vi "display_michelle_visjitter_stopadded_RandCont_Psuedo_FrameClock.vi"() -> ()   [LabVIEW 2019]
uses:
  <vilib>/Analysis/Matrix/Datatypes/RealMatrix.ctl
  <vilib>/Utility/file.llb/Write Delimited Spreadsheet (DBL).vi
  <vilib>/Analysis/Matrix/NI_Matrix.lvlib
panel:
  out "lambda":dbl
  out "maxITI":dbl
  out "minITII":dbl
  out "goEXP":dbl
  out "ArrayTemp3":T1
  out "StimID2":dbl
  out "Contrast":dbl
  out "TimeOutCounter":i32
  out "ElapsedTime_M":dbl
  out "Base_Contrast":dbl
  out "CurrentTrial":u32=1
  out "Jitter":dbl
  out "BaseITI":dbl
  out "VisStimDuration":dbl
  in  "Stop":bool
  out "Num trials":u32=204
  out "ISI Time":dbl
  out "Stim TS":dbl
  out "Output":dbl[][](array[numeric])
  out "Output frame":T1
  out "Array temp1":T1
  out "Elapsed Time":dbl
  out "Display":bool=TRUE
  out "Trial":u32=1
  out "reward":dbl[](array[numeric])
  out "stim_id":dbl[](array[numeric])
  out "stim_loaded":dbl
  out "Timings":dbl[](array[numeric])
  out "Stimuli Loaded?":bool
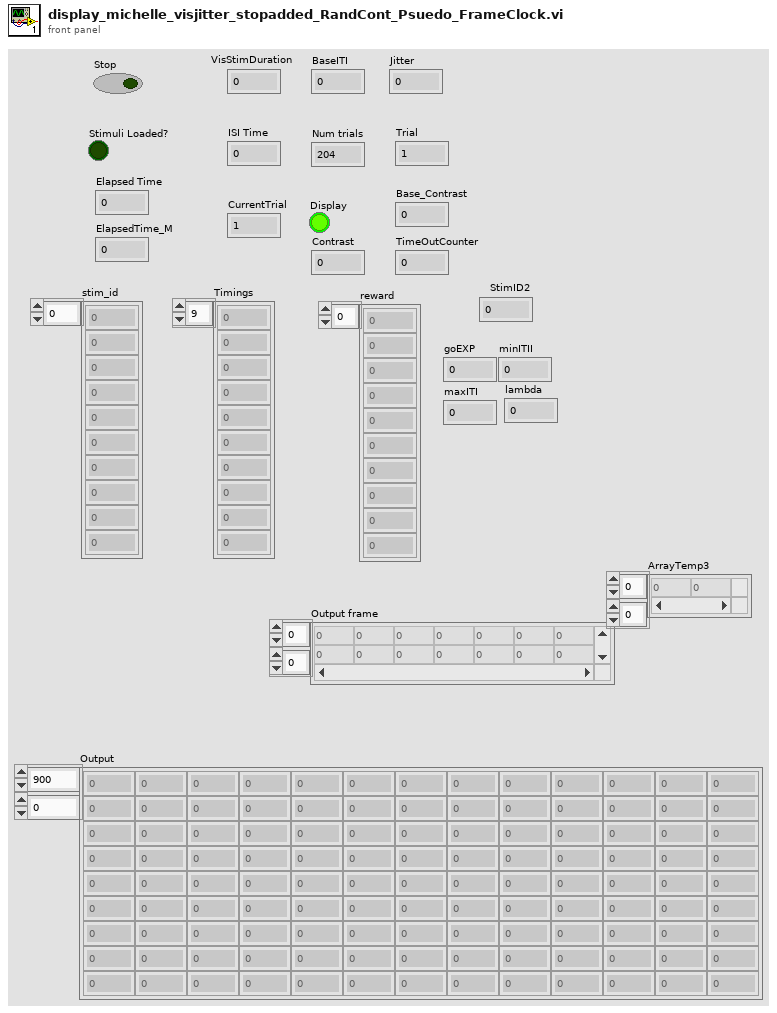
[diagram p1: front panel]
types:
  T1 = typedef "NI_Matrix.lvlib/RealMatrix.ctl" = dbl[][]
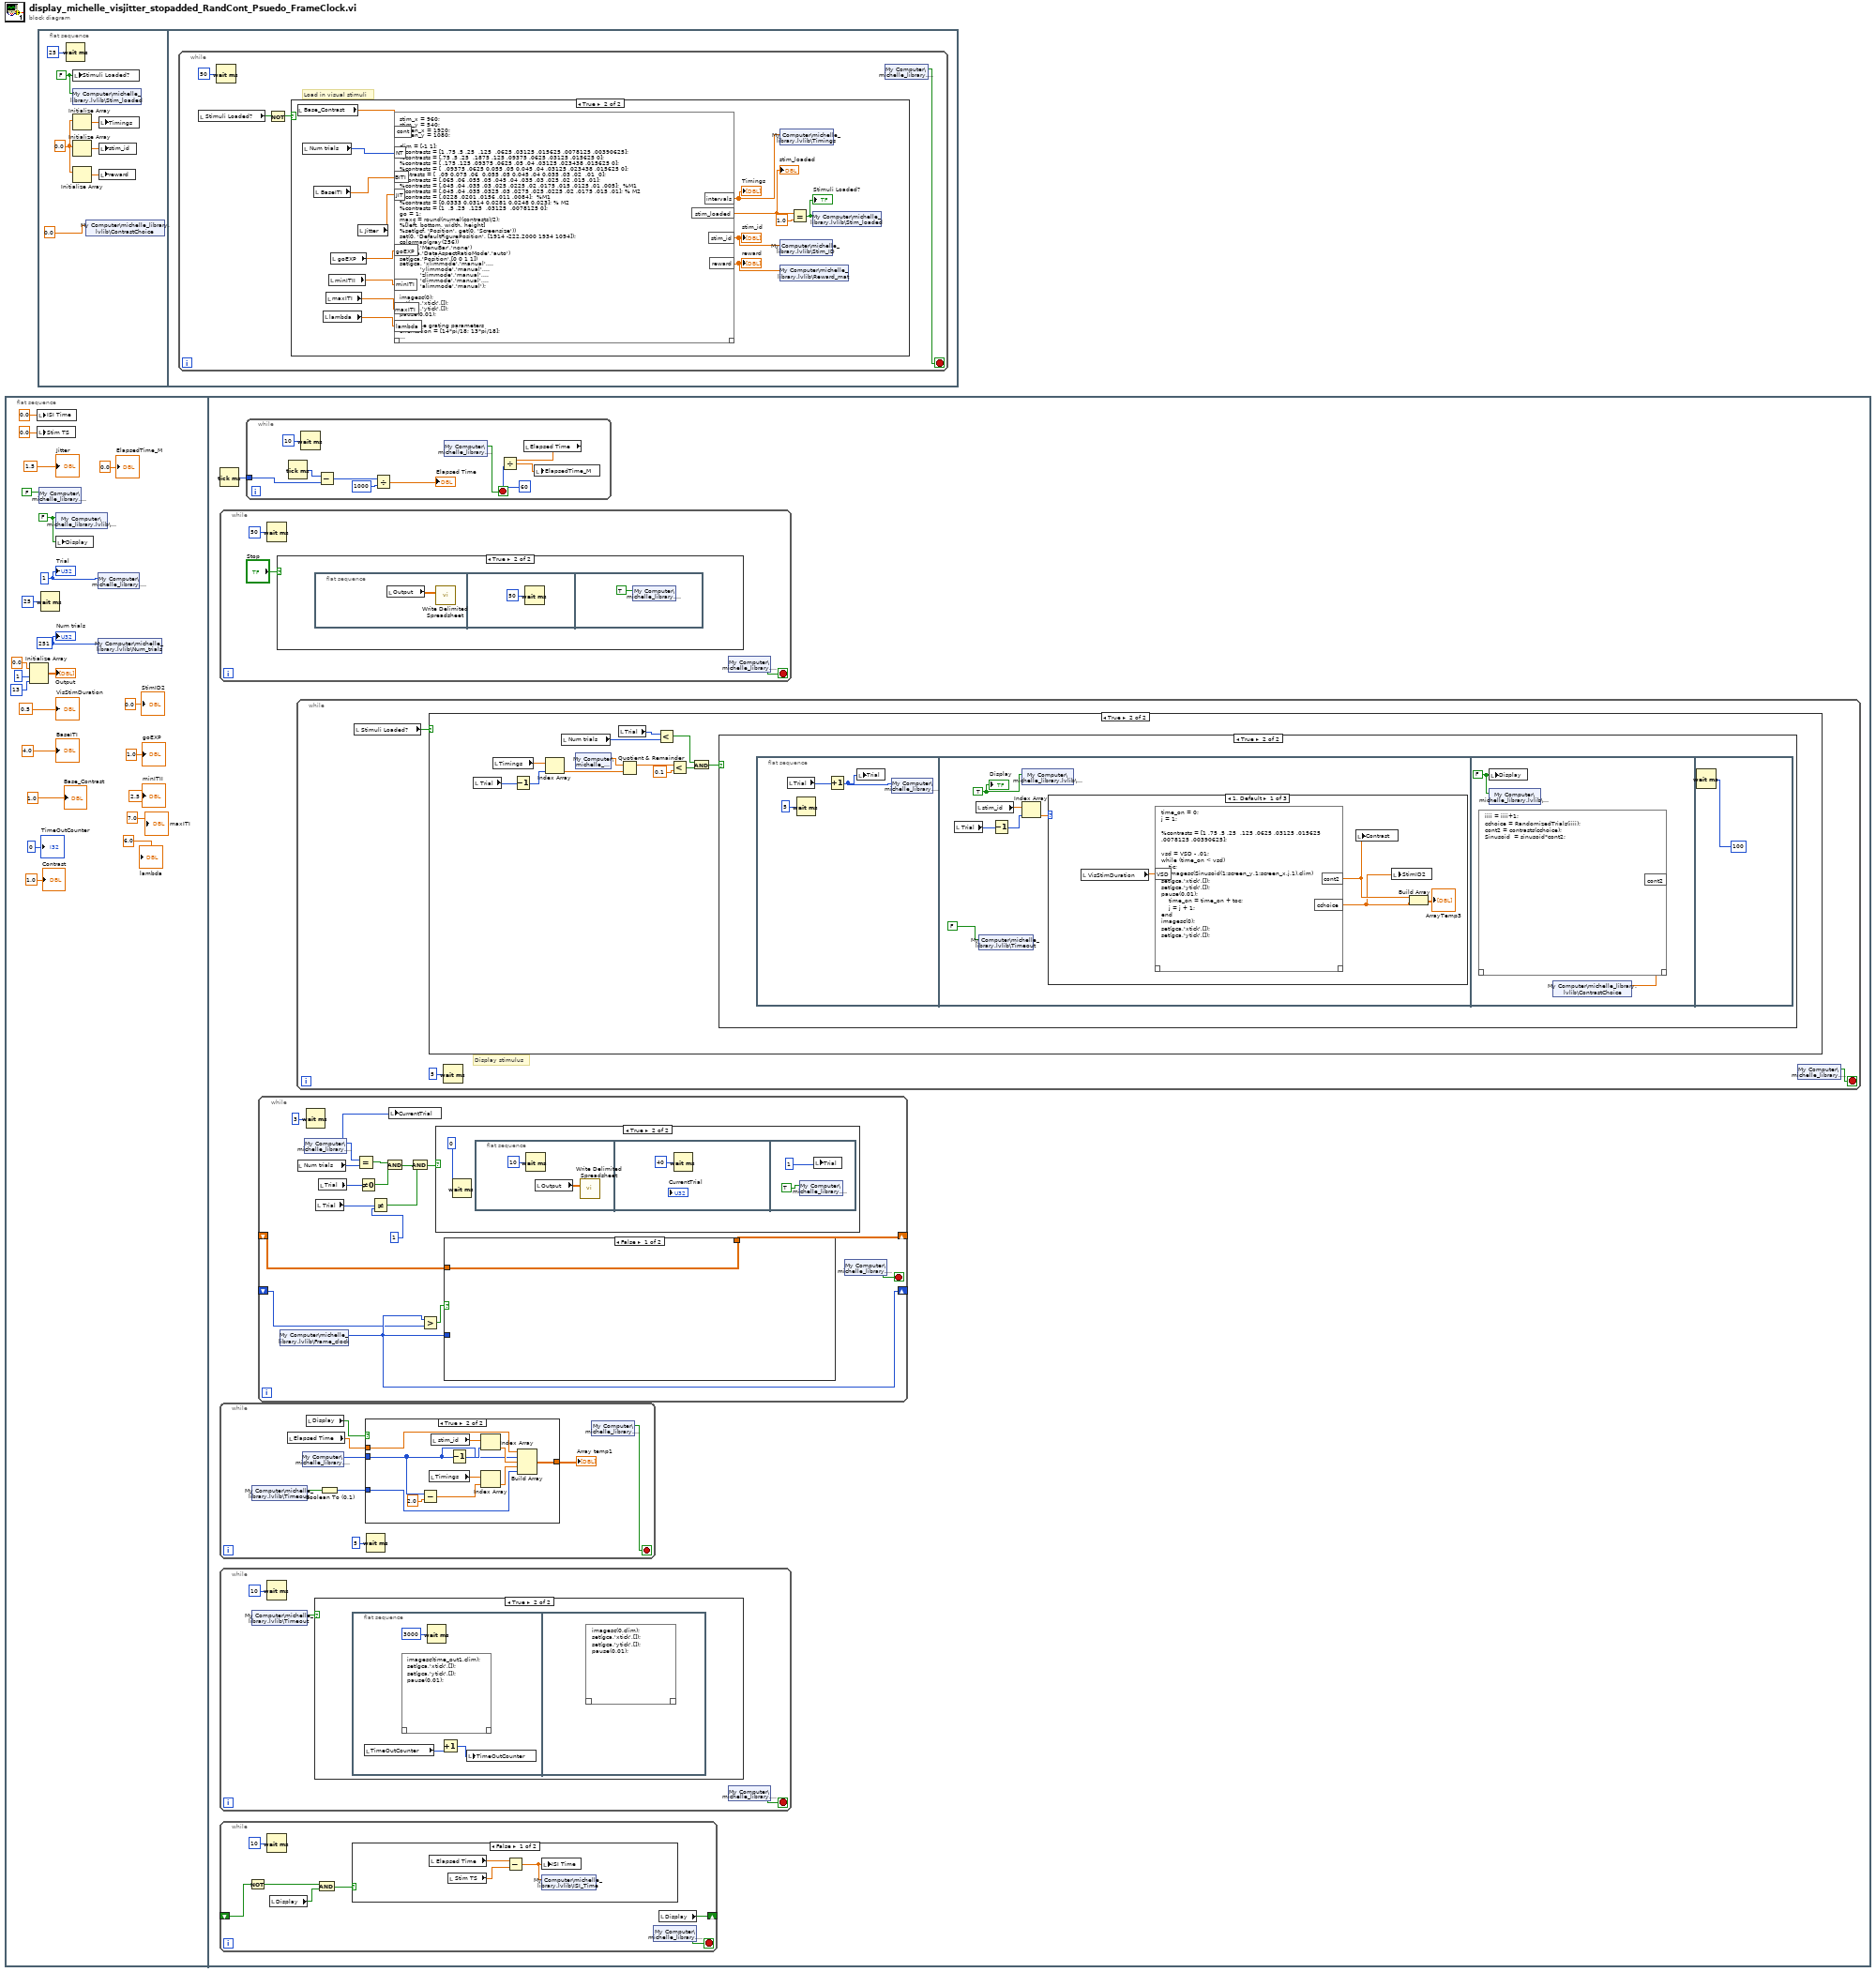
[diagram p0: block diagram]
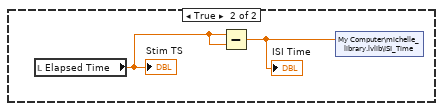
[diagram p5: hidden frame]
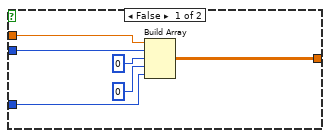
[diagram p6: hidden frame]
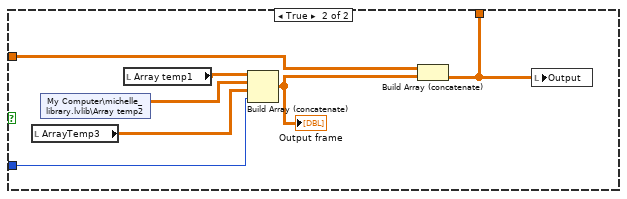
[diagram p7: hidden frame]
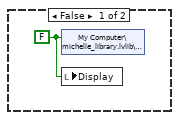
[diagram p10: hidden frame]
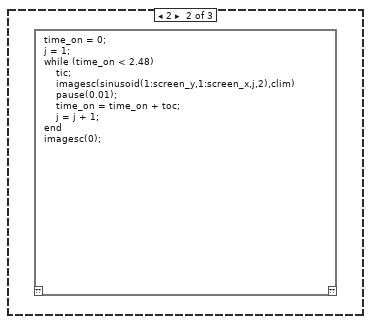
[diagram p11: hidden frame]
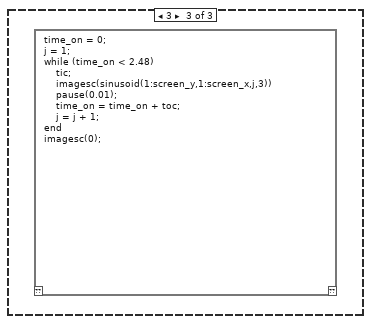
[diagram p12: hidden frame]
diagram:
  n1 = flat-sequence {
    frame #0 {
      w15 = u32 251
      w21 = FALSE ("Display")
      w23 = u32 1 ("Trial")
      n2 = Initialize Array(0.0 ("element"), 1 ("dimension size"), 13 ("dimension size")) -> (→"Output":dbl[][])
      n3 = local write "ISI Time"(0.0 ("ISI Time")) -> ()
      n4 = local write "Stim TS"(0.0 ("Stim TS")) -> ()
      n5 = shared-variable "My Computer\\michelle_library.lvlib\\Stop"(FALSE ("Stop")) -> ()  [unwired: 1 in, 1 out]
      n6 = Wait (ms)(milliseconds to wait=u32 25) -> ()  [unwired: 1 out]
      n7 = shared-variable "My Computer\\michelle_library.lvlib\\Display"(w21) -> ()  [unwired: 1 in, 1 out]
      n8 = local write "Display"(w21) -> ()
      n9 = shared-variable "My Computer\\michelle_library.lvlib\\Trial"(w23) -> ()  [unwired: 1 in, 1 out]
      n10 = shared-variable "My Computer\\michelle_library.lvlib\\Num_trials"(w15) -> ()  [unwired: 1 in, 1 out]
      "Trial" <- w23
      "Num trials" <- w15
      "VisStimDuration" <- 0.5
      "BaseITI" <- 4.0
      "Jitter" <- 1.5
      "Base_Contrast" <- 1.0
      "ElapsedTime_M" <- 0.0
      "TimeOutCounter" <- 0
      "Contrast" <- 1.0
      "StimID2" <- 0.0
      "goEXP" <- 1.0
      "minITII" <- 2.5
      "maxITI" <- 7.0
      "lambda" <- 6.0
    }
    frame #1 {
      n11 = Tick Count (ms)() -> (millisecond timer value=w24:u32)
      n12 = while {
        stop <- w27 stop-if-true
        n13 = Wait (ms)(milliseconds to wait=50) -> ()  [unwired: 1 out]
        n14 = case shown="True" "Stop" {
          frame False {
          }
          frame True {
            n15 = flat-sequence {
              frame #0 {
                n16 = local read "Output"() -> (w28:dbl[][])
                n17 = call-poly <vilib>:"Write Delimited Spreadsheet.vi"("2D data"=w28) -> ()  [unwired: 13 in, 2 out]
              }
              frame #1 {
                n18 = Wait (ms)(milliseconds to wait=50) -> ()  [unwired: 1 out]
              }
              frame #2 {
                n19 = shared-variable "My Computer\\michelle_library.lvlib\\Stop"(TRUE) -> ()  [unwired: 1 in, 1 out]
              }
            }
          }
        }
        n20 = shared-variable "My Computer\\michelle_library.lvlib\\Stop"() -> (w27:bool)  [unwired: 1 in, 1 out]
      }
      n21 = while {
        stop <- w51 stop-if-true
        n22 = shared-variable "My Computer\\michelle_library.lvlib\\Timeout"() -> (w49:bool)  [unwired: 1 in, 1 out]
        n23 = local read "Elapsed Time"() -> (w55:dbl)
        n24 = shared-variable "My Computer\\michelle_library.lvlib\\Trial"() -> (w53:u32)  [unwired: 1 in, 1 out]
        n25 = local read "Display"() -> (w52:bool)
        n26 = Boolean To (0,1)(Boolean=w49) -> (0, 1=w50:i16)
        n27 = case shown="True" w52 {
          tunnel: w53 -> [w61 w64]
          tunnel: w55 -> [w62 w71]
          tunnel: [w60 w72] -> w54
          tunnel: w50 -> [w57 w66]
          frame False {
            n28 = Build Array(w62, w61, u32 0 ("milliseconds to wait"), 0, w57) -> (w60:T1)
          }
          frame True {
            n29 = Subtract(x=w64, y=2.0) -> (x-y=w63:dbl)
            n30 = local read "Timings"() -> (w69:dbl[])
            n31 = local read "stim_id"() -> (w73:dbl[])
            n32 = Decrement(x=w64) -> (x-1=w68:u32)
            n33 = Index Array(array=w73, index=w68) -> (element=w70:dbl)
            n34 = Index Array(array=w69, index=w63) -> (element=w67:dbl)
            n35 = Build Array(w71, w64, w70, w67, w66) -> (w72:T1)
          }
        }
        "Array temp1" <- w54
        n36 = Wait (ms)(milliseconds to wait=u32 5) -> ()  [unwired: 1 out]
        n37 = shared-variable "My Computer\\michelle_library.lvlib\\Stop"() -> (w51:bool)  [unwired: 1 in, 1 out]
      }
      n38 = while {
        stop <- w33 stop-if-true
        n39 = shared-variable "My Computer\\michelle_library.lvlib\\Timeout"() -> (w31:bool)  [unwired: 1 in, 1 out]
        n40 = Wait (ms)(milliseconds to wait=u32 10) -> ()  [unwired: 1 out]
        n41 = case shown="True" w31 {
          frame False {
          }
          frame True {
            n42 = flat-sequence {
              frame #0 {
                n43 = local read "TimeOutCounter"() -> (w35:i32)
                n44 = script code="imagesc(time_out1,clim);\nset(gca,'xtick',[]);\nset(gca,'ytick',[]);\npause(0.01);"() -> ()  [unwired: 1 in, 1 out]
                n45 = Wait (ms)(milliseconds to wait=u32 3000) -> ()  [unwired: 1 out]
                n46 = Increment(x=w35) -> (x+1=w34:i32)
                n47 = local write "TimeOutCounter"(w34) -> ()
              }
              frame #1 {
                n48 = script code="imagesc(0,clim);\nset(gca,'xtick',[]);\nset(gca,'ytick',[]);\npause(0.01);"() -> ()  [unwired: 1 in, 1 out]
              }
            }
          }
        }
        n49 = shared-variable "My Computer\\michelle_library.lvlib\\Stop"() -> (w33:bool)  [unwired: 1 in, 1 out]
      }
      n50 = while {
        shift-right: [w41] -> _
        shift-left: _ -> [w40]
        stop <- w43 stop-if-true
        n51 = Not(x=w40) -> (.not. x?=w39:bool)
        n52 = Wait (ms)(milliseconds to wait=u32 10) -> ()  [unwired: 1 out]
        n53 = local read "Display"() -> (w38:bool)
        n54 = And(x=w39, y=w38) -> (x .and. y?=w37:bool)
        n55 = case shown="False" w37 {
          frame False {
            n56 = local read "Elapsed Time"() -> (w44:dbl)
            n57 = local read "Stim TS"() -> (w46:dbl)
            n58 = Subtract(x=w44, y=w46) -> (x-y=w45:dbl)
            n59 = local write "ISI Time"(w45) -> ()
            n60 = shared-variable "My Computer\\michelle_library.lvlib\\ISI_Time"(w45) -> ()  [unwired: 1 in, 1 out]
          }
          frame True {
            n61 = local read "Elapsed Time"() -> (w47:dbl)
            "Stim TS" <- w47
            n62 = Subtract(x=w47, y=w47) -> (x-y=w48:dbl)
            "ISI Time" <- w48
            n63 = shared-variable "My Computer\\michelle_library.lvlib\\ISI_Time"(w48) -> ()  [unwired: 1 in, 1 out]
          }
        }
        n64 = shared-variable "My Computer\\michelle_library.lvlib\\Stop"() -> (w43:bool)  [unwired: 1 in, 1 out]
        n65 = local read "Display"() -> (w41:bool)
      }
      n66 = while {
        tunnel: w24 -> [w80]
        stop <- w77 stop-if-true
        n67 = Tick Count (ms)() -> (millisecond timer value=w81:u32)
        n68 = Wait (ms)(milliseconds to wait=u32 10) -> ()  [unwired: 1 out]
        n69 = Subtract(x=w81, y=w80) -> (x-y=w78:u32)
        n70 = Divide(x=w78, y=u32 1000) -> (x/y=→"Elapsed Time":dbl)
        n71 = shared-variable "My Computer\\michelle_library.lvlib\\Stop"() -> (w77:bool)  [unwired: 1 in, 1 out]
        n72 = local read "Elapsed Time"() -> (w74:dbl)
        n73 = Divide(x=w74, y=60) -> (x/y=w76:dbl)
        n74 = local write "ElapsedTime_M"(w76) -> ()
      }
      n75 = while {
        shift-right: [w97] -> _
        shift-left: _ -> [w98]
        shift-right: [w87] -> _
        shift-left: _ -> [w86]
        stop <- w100 stop-if-true
        n76 = shared-variable "My Computer\\michelle_library.lvlib\\Frame_clock"() -> (w87:u32)  [unwired: 1 in, 1 out]
        n77 = local read "Num trials"() -> (w96:u32)
        n78 = shared-variable "My Computer\\michelle_library.lvlib\\Trial"() -> (w88:u32)  [unwired: 1 in, 1 out]
        n79 = Wait (ms)(milliseconds to wait=u32 3) -> ()  [unwired: 1 out]
        n80 = local read "Trial"() -> (w93:u32)
        n81 = local read "Trial"() -> (w94:u32)
        n82 = Equal?(x=w88, y=w96) -> (x = y?=w95:bool)
        n83 = Not Equal To 0?(x=w94) -> (x != 0?=w91:bool)
        n84 = Not Equal?(x=w93, y=1) -> (x != y?=w92:bool)
        n85 = And(x=w95, y=w91) -> (x .and. y?=w89:bool)
        n86 = local write "CurrentTrial"(w88) -> ()
        n87 = And(x=w89, y=w92) -> (x .and. y?=w90:bool)
        n88 = Greater?(x=w87, y=w86) -> (0:w84:bool)
        n89 = case shown="True" w90 {
          frame False {
          }
          frame True {
            n90 = Wait (ms)(milliseconds to wait=0) -> ()  [unwired: 1 out]
            n91 = flat-sequence {
              frame #0 {
                n92 = Wait (ms)(milliseconds to wait=u32 10) -> ()  [unwired: 1 out]
                n93 = local read "Output"() -> (w111:dbl[][])
                n94 = call-poly <vilib>:"Write Delimited Spreadsheet.vi"("2D data"=w111) -> ()  [unwired: 13 in, 2 out]
              }
              frame #1 {
                n95 = Wait (ms)(milliseconds to wait=u32 40) -> ()  [unwired: 1 out]
              }
              frame #2 {
                n96 = shared-variable "My Computer\\michelle_library.lvlib\\Stop"(TRUE) -> ()  [unwired: 1 in, 1 out]
                n97 = local write "Trial"(1) -> ()
              }
            }
          }
        }
        n98 = case shown="False" w84 {
          tunnel: w98 -> [w101 w108]
          tunnel: [w101 w107] -> w97
          tunnel: w87 -> [_ w102]
          frame False {
          }
          frame True {
            n99 = local read "ArrayTemp3"() -> (w103:T1)
            n100 = shared-variable "My Computer\\michelle_library.lvlib\\Array temp2"() -> (w105:dbl[][])  [unwired: 1 in, 1 out]
            n101 = local read "Array temp1"() -> (w106:T1)
            n102 = Build Array (concatenate)(w106, w105, w103, w102) -> (w104:T1)
            "Output frame" <- w104
            n103 = Build Array (concatenate) ("Build Matrix")(w108, w104) -> (w107:T1)
            n104 = local write "Output"(w107) -> ()
          }
        }
        n105 = shared-variable "My Computer\\michelle_library.lvlib\\Stop"() -> (w100:bool)  [unwired: 1 in, 1 out]
      }
      n106 = while {
        stop <- w116 stop-if-true
        # "Display stimulus"
        n107 = local read "Stimuli Loaded?"() -> (w115:bool)
        n108 = case shown="True" w115 {
          frame False {
          }
          frame True {
            n109 = local read "Trial"() -> (w118:u32)
            n110 = local read "Timings"() -> (w127:dbl[])
            n111 = Decrement(x=w118) -> (x-1=w119:u32)
            n112 = Index Array(array=w127, index=w119) -> (element=w126:dbl)
            n113 = local read "Num trials"() -> (w122:u32)
            n114 = shared-variable "My Computer\\michelle_library.lvlib\\ISI"() -> (w121:dbl)  [unwired: 1 in, 1 out]
            n115 = local read "Trial"() -> (w125:u32)
            n116 = Quotient & Remainder(x=w121, y=w126) -> (x-y*floor(x/y)=w129:dbl)  [unwired: 1 out]
            n117 = Less?(x=w125, y=w122) -> (x < y?=w124:bool)
            n118 = Less?(x=w129, y=0.1) -> (x < y?=w123:bool)
            n119 = And(x=w124, y=w123) -> (x .and. y?=w120:bool)
            n120 = case shown="True" w120 {
              frame False {
                w130 = FALSE ("Display")
                n121 = shared-variable "My Computer\\michelle_library.lvlib\\Display"(w130) -> ()  [unwired: 1 in, 1 out]
                n122 = local write "Display"(w130) -> ()
              }
              frame True {
                n123 = flat-sequence {
                  frame #0 {
                    n124 = local read "Trial"() -> (w133:u32)
                    n125 = Wait (ms)(milliseconds to wait=u32 5) -> ()  [unwired: 1 out]
                    n126 = Increment(x=w133) -> (x+1=w132:u32)
                    n127 = local write "Trial"(w132) -> ()
                    n128 = shared-variable "My Computer\\michelle_library.lvlib\\Trial"(w132) -> ()  [unwired: 1 in, 1 out]
                  }
                  frame #1 {
                    w138 = TRUE ("Boolean")
                    n129 = local read "Trial"() -> (w136:u32)
                    n130 = local read "stim_id"() -> (w139:dbl[])
                    n131 = shared-variable "My Computer\\michelle_library.lvlib\\Timeout"(FALSE) -> ()  [unwired: 1 in, 1 out]
                    n132 = Decrement(x=w136) -> (x-1=w135:u32)
                    n133 = shared-variable "My Computer\\michelle_library.lvlib\\Display"(w138) -> ()  [unwired: 1 in, 1 out]
                    n134 = Index Array(array=w139, index=w135) -> (element=w137:dbl)
                    n135 = case shown="1, Default" w137 {
                      frame 1, Default {
                        n136 = local read "VisStimDuration"() -> (w143:dbl)
                        n137 = script code="time_on = 0;\nj = 1;\n\n%contrasts = [1 .75 .5 .25  .125 .0625 .03125 .015625 .0078125 .00390625];\n\nvsd = VSD - .01;\nwhile (time_on < vsd)\n    tic;\n    imagesc(Sinusoid(1:screen_y,1:screen_x,j,1),clim)\nset(gca,'xtick',[]);\nset(gca,'ytick',[]);    \npause(0.01);\n    time_on = time_on + toc;\n    j = j + 1;\nend\nimagesc(0);\nset(gca,'xtick',[]);\nset(gca,'ytick',[]);"("VSD"=w143) -> ("cont2"=w142:dbl, "cchoice"=w141:dbl)  [unwired: 1 in, 1 out]
                        n138 = local write "Contrast"(w142) -> ()
                        n139 = local write "StimID2"(w141) -> ()
                        n140 = Build Array(w142, w141) -> (→"ArrayTemp3":T1)
                      }
                      frame 2 {
                        n141 = script code="time_on = 0;\nj = 1;\nwhile (time_on < 2.48)\n    tic;\n    imagesc(sinusoid(1:screen_y,1:screen_x,j,2),clim)\n    pause(0.01);\n    time_on = time_on + toc;\n    j = j + 1;\nend\nimagesc(0);"() -> ()  [unwired: 1 in, 1 out]
                      }
                      frame 3 {
                        n142 = script code="time_on = 0;\nj = 1;\nwhile (time_on < 2.48)\n    tic;\n    imagesc(sinusoid(1:screen_y,1:screen_x,j,3))\n    pause(0.01);\n    time_on = time_on + toc;\n    j = j + 1;\nend\nimagesc(0);"() -> ()  [unwired: 1 in, 1 out]
                      }
                    }
                    "Display" <- w138
                  }
                  frame #2 {
                    w145 = FALSE ("Display")
                    n143 = script code="iiii = iiii+1;\ncchoice = RandomizedTrials(iiii);\ncont2 = contrasts(cchoice);\nSinusoid  = sinusoid*cont2;"() -> ("cont2"=w144:dbl)  [unwired: 1 in, 1 out]
                    n144 = local write "Display"(w145) -> ()
                    n145 = shared-variable "My Computer\\michelle_library.lvlib\\Display"(w145) -> ()  [unwired: 1 in, 1 out]
                    n146 = shared-variable "My Computer\\michelle_library.lvlib\\ContrastChoice"(w144) -> ()  [unwired: 1 in, 1 out]
                  }
                  frame #3 {
                    n147 = Wait (ms)(milliseconds to wait=u32 100) -> ()  [unwired: 1 out]
                  }
                }
              }
            }
          }
        }
        n148 = Wait (ms)(milliseconds to wait=u32 5) -> ()  [unwired: 1 out]
        n149 = shared-variable "My Computer\\michelle_library.lvlib\\Stop"() -> (w116:bool)  [unwired: 1 in, 1 out]
      }
    }
  }
  n150 = flat-sequence {
    frame #0 {
      w150 = 0.0 ("element")
      w148 = FALSE ("Stimuli Loaded?")
      n151 = Wait (ms)(milliseconds to wait=u32 25) -> ()  [unwired: 1 out]
      n152 = local write "Stimuli Loaded?"(w148) -> ()
      n153 = shared-variable "My Computer\\michelle_library.lvlib\\Stim_loaded"(w148) -> ()  [unwired: 1 in, 1 out]
      n154 = Initialize Array(w150) -> (w152:dbl[])  [unwired: 1 in]
      n155 = Initialize Array(w150) -> (w151:dbl[])  [unwired: 1 in]
      n156 = Initialize Array(w150) -> (w149:dbl[])  [unwired: 1 in]
      n157 = shared-variable "My Computer\\michelle_library.lvlib\\ContrastChoice"(0.0) -> ()  [unwired: 1 in, 1 out]
      n158 = local write "Timings"(w152) -> ()
      n159 = local write "stim_id"(w151) -> ()
      n160 = local write "reward"(w149) -> ()
    }
    frame #1 {
      n161 = while {
        stop <- w156 stop-if-true
        # "Load in visual stimuli"
        n162 = local read "Stimuli Loaded?"() -> (w155:bool)
        n163 = Wait (ms)(milliseconds to wait=u32 50) -> ()  [unwired: 1 out]
        n164 = Not(x=w155) -> (.not. x?=w154:bool)
        n165 = case shown="True" w154 {
          frame False {
          }
          frame True {
            n166 = local read "Base_Contrast"() -> (w162:dbl)
            n167 = local read "Num trials"() -> (w165:u32)
            n168 = local read "BaseITI"() -> (w164:dbl)
            n169 = local read "lambda"() -> (w161:dbl)
            n170 = local read "maxITI"() -> (w160:dbl)
            n171 = local read "minITII"() -> (w159:dbl)
            n172 = local read "goEXP"() -> (w158:dbl)
            n173 = local read "Jitter"() -> (w163:dbl)
            n174 = script code="stim_x = 960;\nstim_y = 540;\nscreen_x = 1920;\nscreen_y = 1080;\n\nclim = [-1 1];\n%contrasts = [1 .75 .5 .25  .125  .0625 .03125 .015625 .0078125 .00390625];\n%contrasts = [.75 .5 .25  .1875 .125 .09375 .0625 .03125 .015625 0];\n%contrasts = [ .175 .125 .09375 .0625 .05 .04 .03125 .023438 .015625 0];\n%contrasts = [  .09375 .0625 0.055 .05 0.045 .04 .03125 .023438 .015625 0];\ncontrasts = [  .09 0.075 .06  0.055 .05 0.045 .04 0.035 .03 .02  .01  0];\n%contrasts = [.065 .06 .055 .05 .045 .04 .035 .03 .025 .02 .015 .01];\n%contrasts = [.045 .04 .035 .03 .025 .0225 .02 .0175 .015 .0125 .01 .005];  %M1\n%contrasts = [.045 .04 .035 .0325 .03 .0275 .025 .0225 .02 .0175 .015 .01]; % M2\n%contrasts = [.0228 .0201 .0156 .011 .0084];  %M1\n%contrasts = [0.0333 0.0314 0.0281 0.0248 0.023]; % M2\n%contrasts = [1  .5 .25  .125  .03125  .0078125 0];\ngo = 1;\nmaxc = round(numel(contrasts)/2);\n%[left, bottom, width, height]\n%set(gcf, 'Position', get(0, 'Screensize'))\nset(0, 'DefaultFigurePosition', [1914 -222.2000 1934 1094]);\ncolormap(gray(256))\nset(gcf,'MenuBar','none')\nset(gca,'DataAspectRatioMode','auto')\nset(gca,'Position',[0 0 1 1])\nset(gca, 'xlimmode','manual',...\n           'ylimmode','manual',...\n           'zlimmode','manual',...\n           'climmode','manual',...\n           'alimmode','manual');\n\nimagesc(0);\nset(gca,'xtick',[]);\nset(gca,'ytick',[]);\npause(0.01);\n\n% Define grating parameters\norientation = [14*pi/18; 13*pi/18];\n\ncenter = [1,1]; %[0,0] is the middle of the image, [pi,pi] is the lower right\n%width = .5;  %1/e half width of Gaussian\nspatialFrequency = 8;  %spatial frequency of Sinewave carrier (cycles/image)\nphase = -pi/2; %spatial phase of sinewave carrier (radians)\ncontrast = cont;  %contrast ranges from 0 to 1;\n%screen_x = 1920; %resolution of the image  \n%screen_y = 1080;\n\n% Use meshgrid to define matrices X and Y that range from -pi to pi;\n[X,Y] = meshgrid(linspace(-pi,pi,screen_x),linspace(-pi/2,pi/2,screen_y));\n\nsinusoid = zeros(screen_y,screen_x,150,2);\ntime_out1 = ones(screen_y,screen_x)*-1;\ntime_out2 = zeros(screen_y,screen_x);\n%time_out(1,1) = 1;\n% Set up individual 4-d matrices (x, y, time, orientation) for movies of the drifting gratings at each\n% orientation\nfor j = 1:length(orientation)                                                            % Phase increase number here\n    ramp(1:screen_y,1:screen_x,j) = cos(orientation(j))*(X-center(1)) + sin(orientation(j))*(Y-center(2));     %  |\n    for i = 1:150 %Sets the number of frames to define gratings for                   V\n       sinusoid(1:screen_y,1:screen_x,i,j) = contrast*sin(spatialFrequency*ramp(1:screen_y,1:screen_x,j)-...\n           (phase+(2*pi*(i-1)*(-30)/360))); %Number before '/360' sets the phase increase\n    end\nend\n\n\n\n[RandomizedTrials]=RandomizeTrials_Psuedo_function(contrasts,NT,'n');\n\n\niiii = 1;\n\ncchoice = RandomizedTrials(iiii);\ncont2 = contrasts(cchoice);\nSinusoid  = sinusoid*cont2;\n\n\n%%  To be run of not using exponential\n%intervals = [ones(1,41)*10 ones(1,41)*11 ones(1,41)*12 ones(1,41)*13 ones(1,40)*14];\nif goEXP < 1\n     jit = JIT;\n     jitter = rand(1,NT);\n     jitter = 2*jit*(jitter- .5);\n     ITIbase = BITI;\n     intervals = [ones(1,NT)*ITIbase];\n     intervals = intervals + jitter;\nelseif goEXP > 0\n     intervals = exponentialITI(1/lambda, minITI, maxITI, NT);\nend\n%%\nstim_id = [ones(1,NT)*1];\n%reward = [ones(1,87)*1 ones(1,15)*0 ones(1,87)*1 ones(1,15)*0];\nreward = [ones(1,NT)*1];\n\n\n\nrand_idx1 = randperm(NT);\nrand_idx2 = randperm(NT);\nintervals = intervals(rand_idx2);\nstim_id = stim_id(rand_idx2);\nreward = reward(rand_idx2);\n\nstim_loaded = 1;" ("Script Node")("NT"=w165, "BITI"=w164, "JIT"=w163, "cont"=w162, "goEXP"=w158, "minITI"=w159, "maxITI"=w160, "lambda"=w161) -> ("stim_loaded"=w171:dbl, "intervals"=w166:dbl[], "stim_id"=w167:dbl[], "reward"=w169:dbl[])  [unwired: 1 in, 1 out]
            "stim_loaded" <- w171
            "Timings" <- w166
            "stim_id" <- w167
            "reward" <- w169
            n175 = shared-variable "My Computer\\michelle_library.lvlib\\Timings"(w166) -> ()  [unwired: 1 in, 1 out]
            n176 = shared-variable "My Computer\\michelle_library.lvlib\\Stim_ID"(w167) -> ()  [unwired: 1 in, 1 out]
            n177 = shared-variable "My Computer\\michelle_library.lvlib\\Reward_mat"(w169) -> ()  [unwired: 1 in, 1 out]
            n178 = Equal?(x=w171, y=1.0) -> (x = y?=w168:bool)
            "Stimuli Loaded?" <- w168
            n179 = shared-variable "My Computer\\michelle_library.lvlib\\Stim_loaded"(w168) -> ()  [unwired: 1 in, 1 out]
          }
        }
        n180 = shared-variable "My Computer\\michelle_library.lvlib\\Stop"() -> (w156:bool)  [unwired: 1 in, 1 out]
      }
    }
  }
